vi "Set Error.vi"(0 "LVx.lvlib:LVx.lvclass":refnum<class "LVx.lvclass">, 11 "error in (no error)":errorcluster) -> (4 "LVx.lvlib:LVx.lvclass 2":refnum<class "LVx.lvclass">, 15 "error out":errorcluster)   [LabVIEW 2011, in "LVx.lvlib" / "LVx.lvclass"]
uses:
  LVx.lvclass
  LVx.lvclass/LVx.ctl
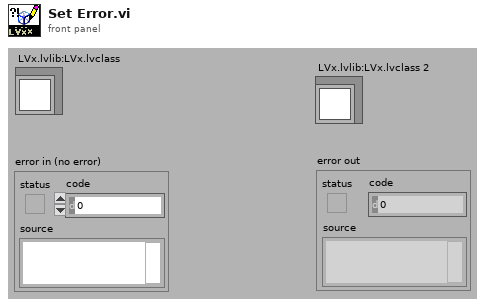
[diagram p1: front panel]
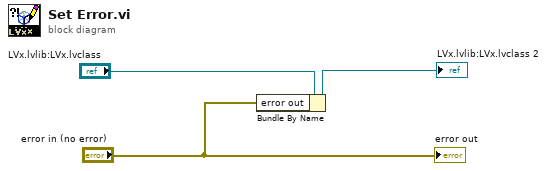
[diagram p0: block diagram]
diagram:
  n1 = Bundle By Name(cluster="LVx.lvlib:LVx.lvclass", "error out"="error in (no error)") -> (→"LVx.lvlib:LVx.lvclass 2":refnum<class "LVx.lvclass">)
  "error out" <- "error in (no error)"
